vi "Get Subpackets.vi"(8 "error in (no error)":errorcluster, 11 "Operator in":refnum<class "Operator.lvclass">) -> (0 "error out":errorcluster, 2 "Subpackets":refnum<class "Packet.lvclass">[](array[class]), 3 "Operator out":refnum<class "Operator.lvclass">)   [LabVIEW 2020, in "Operator.lvclass"]
uses:
  Operator.lvclass
  Packet/Packet.lvclass
  Operator.lvclass/Operator.ctl
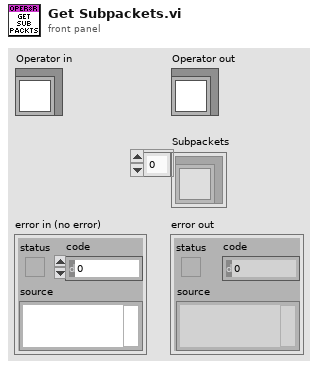
[diagram p1: front panel]
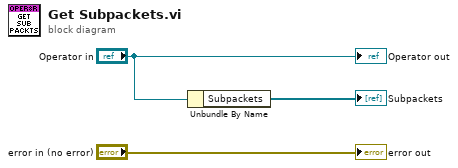
[diagram p0: block diagram]
diagram:
  n1 = Unbundle By Name("Operator in") -> ("Subpackets"=→"Subpackets":refnum<class "Packet.lvclass">[])
  "error out" <- "error in (no error)"
  "Operator out" <- "Operator in"
